vi "Check Responses.vi"(10 "delays":u16[](array[numeric]), 11 "responses":T1[](array[typedef])) -> (0 "consecutive requests?":bool, 1 "delays match?":bool, 2 "response delays":u16[](array[numeric]))   [LabVIEW 2023]
uses:
  <instrlib>/niUSRP/Reference FPGA/ZBX Control/ZBX IO Response.ctl
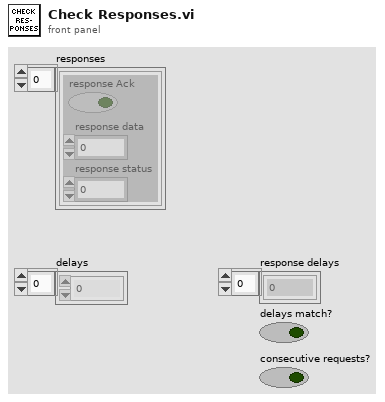
[diagram p1: front panel]
types:
  T1 = typedef "ZBX IO Response.ctl" = cluster{"response Ack":bool, "response data":u32, "response status":fxp<+,2,2>}
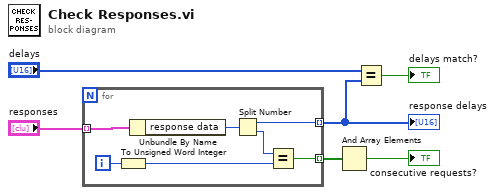
[diagram p0: block diagram]
diagram:
  n1 = for {
    tunnel: "responses" -> [w13] mode=indexing
    tunnel: [w11] -> w3 mode=indexing
    tunnel: [w7] -> w2 mode=indexing
    i -> [w8]
    n2 = To Unsigned Word Integer(number=w8) -> (unsigned 16bit integer=w9:u16)
    n3 = Unbundle By Name(w13) -> ("response data"=w12:u32)
    n4 = Split Number(x=w12) -> (hi(x)=w11:u16, lo(x)=w10:u16)
    n5 = Equal?(x=w10, y=w9) -> (x = y?=w7:bool)
  }
  "response delays" <- w3
  n6 = And Array Elements(Boolean array=w2) -> (logical AND=→"consecutive requests?":bool)
  n7 = Equal?(x="delays", y=w3) -> (x = y?=→"delays match?":bool)
